vi "_Start Monitor VI.vi"(8 "error in (no error)":errorcluster) -> (0 "error out":errorcluster)   [LabVIEW 2017]
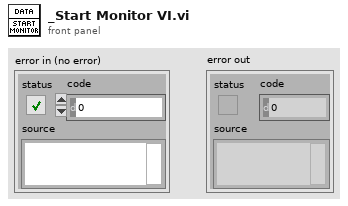
[diagram p1: front panel]
types:
  T1 = enum32{"Bad", "Idle", "Run top level", "Running"}
  T2 = enum32{"Invalid", "Standard", "Closed", "Hidden", "Minimized", "Maximized"}
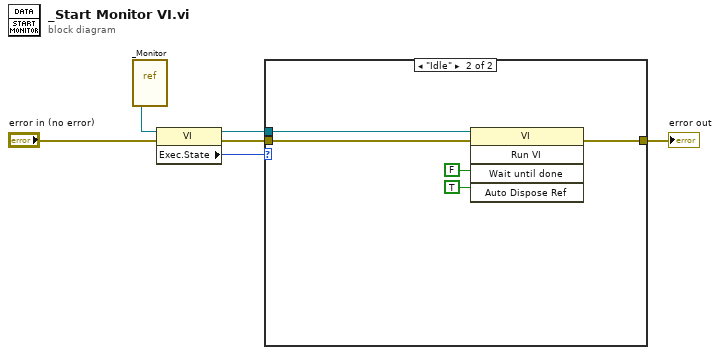
[diagram p0: block diagram]
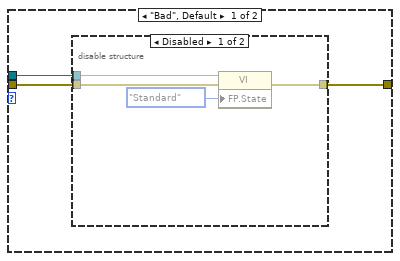
[diagram p2: hidden frame]
diagram:
  n1 = vi-ref "_Monitor.vi"() -> (w6:refnum<vi>)
  n2 = property class="VI"(reference=w6, error in="error in (no error)") -> (reference out=w3:refnum<vi>, error out=w5:errorcluster, "Exec.State"=w4:T1)
  n3 = case shown="\"Idle\"" w4 {
    tunnel: w5 -> [w9 w18]
    tunnel: w3 -> [w7 w19]
    tunnel: [w8 w15] -> w2
    frame "Bad", Default {
      n4 = disable-structure shown="Disabled" {
        disable-tunnel: w9 -> [w13 w14]
        disable-tunnel: [w12 w14] -> w8
        disable-tunnel: w7 -> [w11 _]
        frame Disabled {
          n5 = property class="VI"(reference=w11, error in=w13, "FP.State"=T2."Standard" ("Front Panel Window:State")) -> (error out=w12:errorcluster)  [unwired: 1 out]
        }
        frame Enabled {
        }
      }
    }
    frame "Idle" {
      n6 = invoke class="VI" method="Run VI"(reference=w19, error in=w18, "Wait until done"=FALSE ("Wait Until Done"), "Auto Dispose Ref"=TRUE ("Auto Dispose Reference")) -> (error out=w15:errorcluster)  [unwired: 1 in, 4 out]
    }
  }
  "error out" <- w2
